vi "Read Scale Range Minimum.vi"(6 "Control Ref Queue":T1, 8 "error in (no error)":errorcluster, 9 "Index":i32, 11 "2D Plot.lvclass in":refnum<class "2D Plot.lvclass">) -> (0 "error out":errorcluster, 2 "Minimum":dbl, 3 "2D Plot.lvclass out":refnum<class "2D Plot.lvclass">)   [LabVIEW 2020, in "2D Plot.lvclass"]
uses:
  <vilib>/Math Plots/2D Math Plots/2D Plot/2D Plot/2D Plot.lvclass
  <vilib>/Math Plots/2D Math Plots/2D Plot/Action String/2DMathPlot Ctrl Act Queue.ctl
  <vilib>/Math Plots/2D Math Plots/2D Plot/Action String/2DMathPlot Ctrl Act Cluster.ctl
  <vilib>/Math Plots/2D Math Plots/2D Plot/Action String/2DMathPlot State Class.ctl
  <vilib>/Math Plots/2D Math Plots/2D Plot/2D Plot/2D Plot.lvclass/2D Plot.ctl
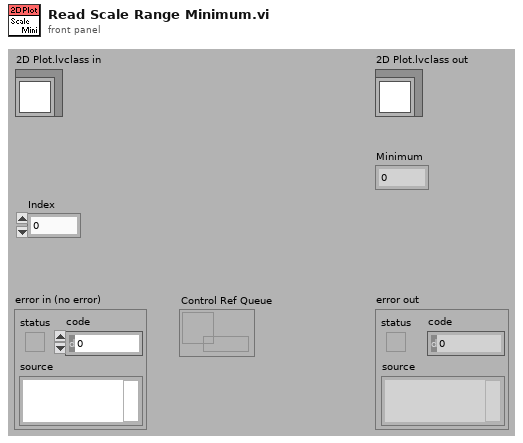
[diagram p1: front panel]
types:
  T1 = typedef "2DMathPlot Ctrl Act Queue.ctl" = refnum<queue>
  T2 = typedef "2DMathPlot Ctrl Act Cluster.ctl" = cluster{"Plot Area Ref":refnum<vi>, "Z Axis Ref":refnum<vi>, "Legend Ref":refnum<vi>, "XControl Ref":refnum<vi>, "Facade Ref":refnum<vi>, "Display State Change Class":T3}
  T3 = typedef "2DMathPlot State Class.ctl" = enum16{"Update All (Undo)", "Update General", "Update Appearance", "Update Format", "Update Scale", "Update Marker", "Update Cursor", "None"}
  T4 = typedef "2D Plot.lvclass/Scale Array.ctl" = T5[]
  T5 = typedef "2D Plot.lvclass/Scale Cluster.ctl" = cluster{"General":cluster{"Editable":bool, "Flipped":bool, "Mapping Mode":u8, "Visible":bool, "Style":u8, "Scale Fit":u8}, "Offset and Multiplier":T6, "Range":cluster{"Minimum":dbl, "Maximum":dbl, "Increment":dbl, "Minor Increment":dbl, "Start":dbl}, "Tick Color":cluster{"Major Color":u32, "Minor Color":u32}, "Gird Color":cluster{"Major Color":u32, "Minor Color":u32}, "Marker":cluster{"Visible":bool, "FG Color":u32, "BG Color":u32, "Font Name":string, "Font Size":u32, "Font Bold":bool, "Font Italic":bool, "Font Strikeout":bool, "Font Underline":bool}, "Name Label":cluster{"Visible":bool, "FG Color":u32, "BG Color":u32, "Font Name":string, "Font Size":u32, "Font Bold":bool, "Font Italic":bool, "Font Strikeout":bool, "Font Underline":bool, "Justification":enum16{"Left", "Center", "Right"}, "Text":string}}
  T6 = typedef "LVOffsetAndMultiplierTypeDef.ctl" = cluster{"Offset":dbl, "Multiplier":dbl}
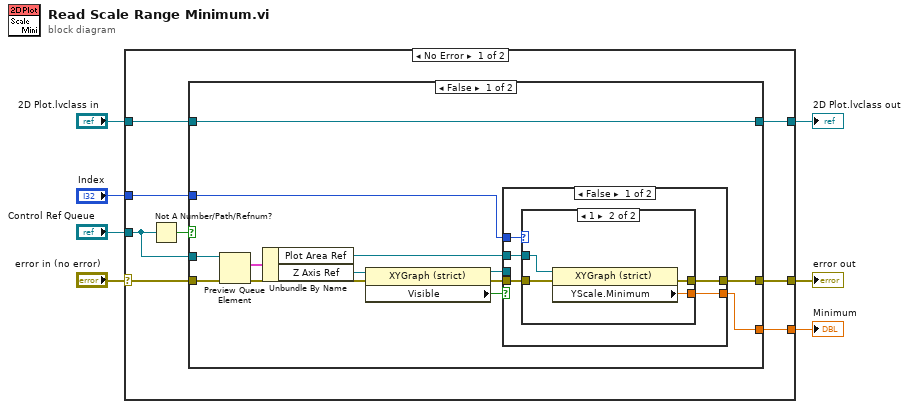
[diagram p0: block diagram]
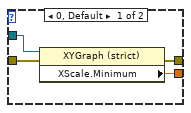
[diagram p2: hidden frame]
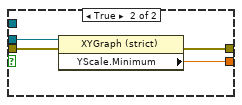
[diagram p3: hidden frame]
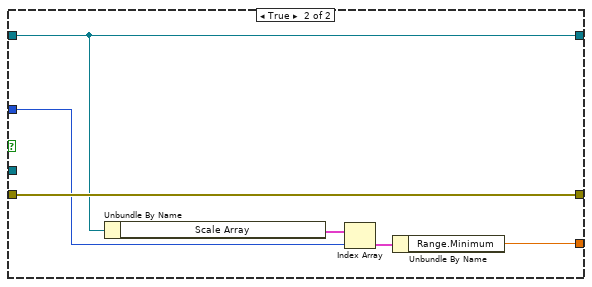
[diagram p4: hidden frame]
diagram:
  n1 = case shown="No Error" "error in (no error)" {
    selector: "error in (no error)" -> [w10 w53]
    tunnel: "Index" -> [w15 _]
    tunnel: [w14 w53] -> w6
    tunnel: [w13 _] -> w5
    tunnel: "Control Ref Queue" -> [w12 _]
    tunnel: "2D Plot.lvclass in" -> [w9 w52]
    tunnel: [w8 w52] -> w1
    frame No Error {
      n2 = Not A Number/Path/Refnum?(number/path/refnum=w12) -> (NaN/Path/Refnum?=w11:bool)
      n3 = case shown="False" w11 {
        tunnel: w15 -> [w22 w47]
        tunnel: w10 -> [w21 w49]
        tunnel: [w20 w49] -> w14
        tunnel: [w19 w48] -> w13
        tunnel: w12 -> [w18 _]
        tunnel: w9 -> [w17 w46]
        tunnel: [w17 w46] -> w8
        frame False {
          n4 = Preview Queue Element(queue=w18, error in (no error)=w21) -> (element=w28:T2, error out=w26:errorcluster)  [unwired: 1 in, 2 out]
          n5 = Unbundle By Name(w28) -> ("Plot Area Ref"=w25:refnum<vi>, "Z Axis Ref"=w16:refnum<vi>)
          n6 = property class="XYGraph (strict)"(reference=w16, error in=w26) -> (reference out=w24:refnum<vi>, error out=w23:errorcluster, "Visible"=w27:bool)
          n7 = case shown="False" w27 {
            tunnel: w22 -> [w33 _]
            tunnel: w23 -> [w32 w42]
            tunnel: [w31 w43] -> w19
            tunnel: [w30 w44] -> w20
            tunnel: w25 -> [w29 _]
            tunnel: w24 -> [_ w45]
            frame False {
              n8 = case shown="1" w33 {
                tunnel: w32 -> [w37 w41]
                tunnel: [w36 w40] -> w30
                tunnel: [w35 w39] -> w31
                tunnel: w29 -> [w34 w38]
                frame 0, Default {
                  n9 = property class="XYGraph (strict)"(reference=w34, error in=w37) -> (error out=w36:errorcluster, "XScale.Minimum"=w35:dbl)  [unwired: 1 out]
                }
                frame 1 {
                  n10 = property class="XYGraph (strict)"(reference=w38, error in=w41) -> (error out=w40:errorcluster, "YScale.Minimum"=w39:dbl)  [unwired: 1 out]
                }
              }
            }
            frame True {
              n11 = property class="XYGraph (strict)"(reference=w45, error in=w42) -> (error out=w44:errorcluster, "YScale.Minimum"=w43:dbl)  [unwired: 1 out]
            }
          }
        }
        frame True {
          n12 = Unbundle By Name(w46) -> ("Scale Array"=w50:T4)
          n13 = Index Array(array=w50, index=w47) -> (element=w51:T5)
          n14 = Unbundle By Name(w51) -> ("Range.Minimum"=w48:dbl)
        }
      }
    }
    frame Error {
    }
  }
  "error out" <- w6
  "Minimum" <- w5
  "2D Plot.lvclass out" <- w1
